vi "Read Dig Chan.vi"() -> ()   [LabVIEW 2021]
doc: "I. Description:\nThis example demonstrates how to read values from one or more digital input channels.\n\nII. Instructions for Running:\n1. Select the digital lines on the DAQ device to be read.\nNote: The array indicator is sized for 8 lines, if using fewer lines, not all elements will be used. Also, if using more lines, use the array index to view elements beyond the first eight lines.\n\nIII. Block Diagram Steps:\n1. Create a Digital Input channel. Use one channel for all lines. You can alternatively use one channel for each line, but then use a different polymorphic version of the DAQmx Read VI.\n2. Call the Start VI to start the task.\n3. Read the digital data in a loop until the user hits the stop button or an error occurs. This read VI reads a single sample of digital data on demand, so no timeout is necessary.\n4. Use the Boolean Array to Number VI to view the values read as a single number\n5. Call the Clear Task VI to clear the Task.\n6. Use the popup dialog box to display an error or warning if any.\n\nIV. I/O Connections Overview:\nMake sure your signal input terminals match the Lines I/O Control. In this case wire your digital signals to the first eight digital lines on your DAQ Device."
uses:
  <vilib>/userdefined/High Color/nirio_resource_hc.ctl
  <vilib>/FPGAPlugInAG/PCIe-7857/niLvFpga_Open_PCIe-7857.vi
  <vilib>/rvi/interface/common/dynamic/niFpgaDynamicAddResources.vi
  <vilib>/Utility/error.llb/Error Cluster From Error Code.vi
  <vilib>/rvi/errors/niLvFpgaAdjustHostInterfaceError.vi
  <vilib>/FPGAPlugInAG/Dynamic/niLvFpga_Close_Dynamic.vi
  <vilib>/rvi/interface/nirviOpenFPGA/nirviOpenFPGA.xnode
  FPGA Bitfiles/lvfpga_FPGATarget_DIO_kUunw4c2SQ8.lvbitx
  DIO.vi
  <vilib>/rvi/interface/nirviReadWriteControl/nirviReadWriteControl.xnode
  <vilib>/rvi/interface/nirviCloseFPGA/nirviCloseFPGA.xnode
  NiFpgaLv.dll
  <vilib>/rvi/interface/Simulation/niFpgaSimulationCallBeginRW.vi
panel:
  out "Boolean Data Read":bool[](array[boolean])
  in  "RIO Resource Name":T1 caption="RIO Device"
  out "Hexadecimal Data Read":u32 format="%x"
  in  "stop":bool
  # "Channel Parameters"
  # "Bits"
  # "0"
  # "1"
  # "2"
  # "3"
  # "4"
  # "5"
  # "6"
  # "7"
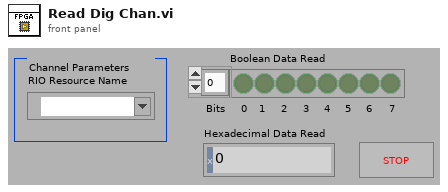
[diagram p1: front panel]
types:
  T1 = typedef "nirio_resource_hc.ctl" = tag
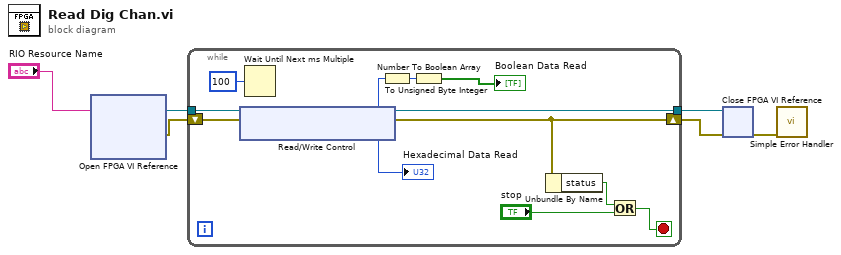
[diagram p0: block diagram]
diagram:
  n1 = xnode "Open FPGA VI Reference"("resource name"="RIO Resource Name") -> ("FPGA VI Reference Out"=w2:refnum<k20>, "error out"=w1:errorcluster)  [unwired: 1 in]
  n2 = while {
    tunnel: w2 -> [w17]
    tunnel: [w15] -> w6
    shift-right: [w12] -> w5
    shift-left: w1 -> [w16]
    stop <- w13 stop-if-true
    n3 = xnode "Read/Write Control"("FPGA VI Reference In"=w17, "error in"=w16) -> ("FPGA VI Reference Out"=w15:refnum<k20>, "error out"=w12:errorcluster, "Connector 1 DIO Port 0"=w9:u8)
    "Hexadecimal Data Read" <- w9
    n4 = Wait Until Next ms Multiple(millisecond multiple=u32 100 ("milliseconds to wait")) -> ()  [unwired: 1 out]
    n5 = To Unsigned Byte Integer(number=w9) -> (unsigned 8bit integer=w8:u8)
    n6 = Number To Boolean Array(number=w8) -> (Boolean array=→"Boolean Data Read":bool[])
    n7 = Unbundle By Name(w12) -> ("status"=w11:bool)
    n8 = Or(x=w11, y="stop") -> (x .or. y?=w13:bool)
  }
  n9 = xnode "Close FPGA VI Reference"("FPGA VI Reference In"=w6, "error in"=w5) -> ("error out"=w4:errorcluster)
  n10 = call <vilib>:"Simple Error Handler.vi"("error in (no error)"=w4) -> ()  [unwired: 4 in, 5 out]
